vi "Generate Value.vi"(10 "base value":i64, 11 "type code":T1=enum."Bool") -> (3 "value":variant)   [LabVIEW 2020]
uses:
  Value/Type Code.ctl
  Value/Value.lvlib
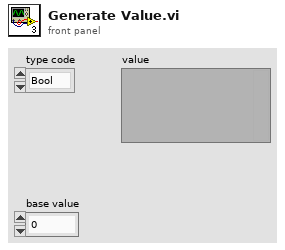
[diagram p1: front panel]
types:
  T1 = typedef "Value.lvlib/Type Code.ctl" = enum8{"Null", "Bool", "BoolA", "Int8", "Int8A", "Int16", "Int16A", "Int32", "Int32A", "Int64", "Int64A", "UInt8", "UInt8A", "UInt16", "UInt16A", "UInt32", "UInt32A", "UInt64", "UInt64A", "Float32", "Float32A", "Float64", "Float64A", "String", "StringA", "Struct", "StructA", "Union", "UnionA", "Any", "AnyA"}
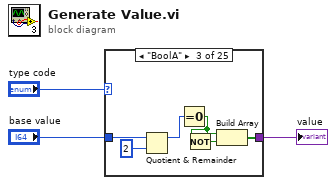
[diagram p0: block diagram]
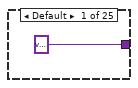
[diagram p2: hidden frame]
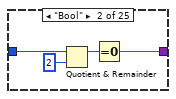
[diagram p3: hidden frame]
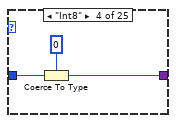
[diagram p4: hidden frame]
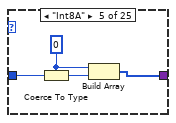
[diagram p5: hidden frame]
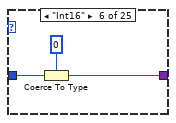
[diagram p6: hidden frame]
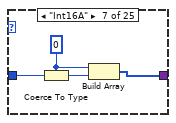
[diagram p7: hidden frame]
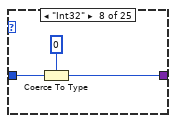
[diagram p8: hidden frame]
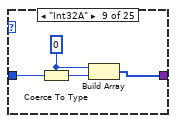
[diagram p9: hidden frame]
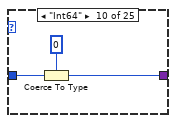
[diagram p10: hidden frame]
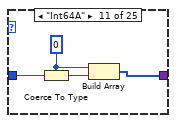
[diagram p11: hidden frame]
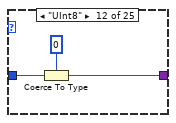
[diagram p12: hidden frame]
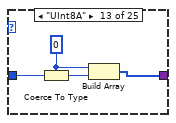
[diagram p13: hidden frame]
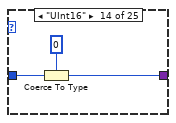
[diagram p14: hidden frame]
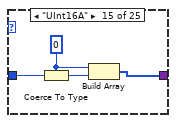
[diagram p15: hidden frame]
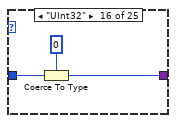
[diagram p16: hidden frame]
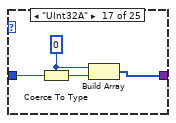
[diagram p17: hidden frame]
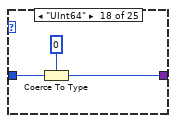
[diagram p18: hidden frame]
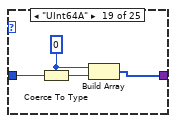
[diagram p19: hidden frame]
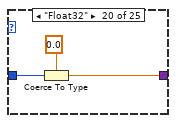
[diagram p20: hidden frame]
diagram:
  n1 = case shown="\"BoolA\"" "type code" {
    tunnel: "base value" -> [_ w7 w12 w16 w21 w24 w28 w31 w35 w38 w42 w45 w49 w52 w56 w59 w63 w66 w70 w73 w76 w80 w84 w86 w90]
    tunnel: [variant w6 w14 w15 w18 w22 w25 w29 w32 w36 w39 w43 w46 w50 w53 w57 w60 w64 w67 w71 w74 w77 w81 w85 w87] -> w1
    frame Default {
    }
    frame "Bool" {
      n2 = Quotient & Remainder(x=w7, y=i64 2) -> (x-y*floor(x/y)=w5:i64)  [unwired: 1 out]
      n3 = Equal To 0?(x=w5) -> (x = 0?=w6:bool)
    }
    frame "BoolA" {
      n4 = Quotient & Remainder(x=w12, y=i64 2) -> (x-y*floor(x/y)=w11:i64)  [unwired: 1 out]
      n5 = Equal To 0?(x=w11) -> (x = 0?=w9:bool)
      n6 = Not(x=w9) -> (.not. x?=w10:bool)
      n7 = Build Array(w9, w10) -> (w14:bool[])
    }
    frame "Int8" {
      n8 = Coerce To Type(0:w16, 1:i8 0 ("default value")) -> (2:w15:i8)
    }
    frame "Int8A" {
      w19 = i8 0 ("default value")
      n9 = Coerce To Type(0:w21, 1:w19) -> (2:w20:i8)
      n10 = Build Array(w19, w20) -> (w18:i8[])
    }
    frame "Int16" {
      n11 = Coerce To Type(0:w24, 1:i16 0 ("default value")) -> (2:w22:i16)
    }
    frame "Int16A" {
      w26 = i16 0 ("default value")
      n12 = Coerce To Type(0:w28, 1:w26) -> (2:w27:i16)
      n13 = Build Array(w26, w27) -> (w25:i16[])
    }
    frame "Int32" {
      n14 = Coerce To Type(0:w31, 1:0 ("default value")) -> (2:w29:i32)
    }
    frame "Int32A" {
      w33 = 0 ("default value")
      n15 = Coerce To Type(0:w35, 1:w33) -> (2:w34:i32)
      n16 = Build Array(w33, w34) -> (w32:i32[])
    }
    frame "Int64" {
      n17 = Coerce To Type(0:w38, 1:i64 0 ("default value")) -> (2:w36:i64)
    }
    frame "Int64A" {
      w40 = i64 0 ("default value")
      n18 = Coerce To Type(0:w42, 1:w40) -> (2:w41:i64)
      n19 = Build Array(w40, w41) -> (w39:i64[])
    }
    frame "UInt8" {
      n20 = Coerce To Type(0:w45, 1:u8 0 ("default value")) -> (2:w43:u8)
    }
    frame "UInt8A" {
      w47 = u8 0 ("default value")
      n21 = Coerce To Type(0:w49, 1:w47) -> (2:w48:u8)
      n22 = Build Array(w47, w48) -> (w46:u8[])
    }
    frame "UInt16" {
      n23 = Coerce To Type(0:w52, 1:u16 0 ("default value")) -> (2:w50:u16)
    }
    frame "UInt16A" {
      w54 = u16 0 ("default value")
      n24 = Coerce To Type(0:w56, 1:w54) -> (2:w55:u16)
      n25 = Build Array(w54, w55) -> (w53:u16[])
    }
    frame "UInt32" {
      n26 = Coerce To Type(0:w59, 1:u32 0 ("default value")) -> (2:w57:u32)
    }
    frame "UInt32A" {
      w61 = u32 0 ("default value")
      n27 = Coerce To Type(0:w63, 1:w61) -> (2:w62:u32)
      n28 = Build Array(w61, w62) -> (w60:u32[])
    }
    frame "UInt64" {
      n29 = Coerce To Type(0:w66, 1:u64 0 ("default value")) -> (2:w64:u64)
    }
    frame "UInt64A" {
      w68 = u64 0 ("default value")
      n30 = Coerce To Type(0:w70, 1:w68) -> (2:w69:u64)
      n31 = Build Array(w68, w69) -> (w67:u64[])
    }
    frame "Float32" {
      n32 = Coerce To Type(0:w73, 1:sgl 0.0 ("default value")) -> (2:w71:sgl)
    }
    frame "Float64" {
      n33 = Coerce To Type(0:w76, 1:0.0 ("default value")) -> (2:w74:dbl)
    }
    frame "Float32A" {
      w78 = sgl 0.0 ("default value")
      n34 = Coerce To Type(0:w80, 1:w78) -> (2:w79:sgl)
      n35 = Build Array(w78, w79) -> (w77:sgl[])
    }
    frame "Float64A" {
      w82 = 0.0 ("default value")
      n36 = Coerce To Type(0:w84, 1:w82) -> (2:w83:dbl)
      n37 = Build Array(w82, w83) -> (w81:dbl[])
    }
    frame "String" {
      n38 = Format Value(value (0)=w86) -> (output string=w85:string)  [unwired: 2 in]
    }
    frame "StringA" {
      n39 = Format Value(value (0)=w90) -> (output string=w89:string)  [unwired: 2 in]
      n40 = Build Array(w89, "Hello" ("element")) -> (w87:string[])
    }
  }
  "value" <- w1
